vi "Impedance_SingleStats.vi"() -> ()   [LabVIEW 2020]
uses:
  <vilib>/Analysis/NI_AALBase.lvlib
panel:
  in  "Current Ch":tag="Dev3/ai1"
  in  "Voltage Ch":tag="Dev3/ai0"
  in  "Output channels":tag="Dev3/ao0"
  in  "TriggerLine":tag="/Dev3/ao/StartTrigger"
  out "Impedance (Phase) - AvgInput":dbl=-0.6720456229115541 format="%#_3p"
  out "Impedance (Mag) - AvgInput":dbl=100001.51067957297 format="%#_3p"
  out "Waveform Chart":dbl(graph)
  in  "Freq":dbl
  out "Histogram Graph Phase":T1(graph)
  out "Histogram Graph Mag":T1(graph)
  out "standard deviation  Z":dbl format="%.2p"
  out "standard deviation Phase":dbl format="%.2p"
  out "Real (Z) - AvgInput":dbl=0.483159362565652 format="%#_3p"
  out "Capacitance - AvgInput":dbl=-4.6875540145244966e-05 format="%#_3p"
  out "Inductance - AvgInput":dbl=5.4037341931629855e-06 format="%#_3p"
  out "Test Number":i32
  in  "Num Avg":i32=5
  out "Mean Phase":dbl format="%0.2f"
  out "Mean Mag":dbl format="%.4p"
  in  "amplitude":dbl=0.1 format="%0.2p"
  in  "SampRate":dbl=250000.0 format="%#.2p"
  in  "Test Time":dbl=1.0 format="%#_6p"
  in  "samples":i32=128
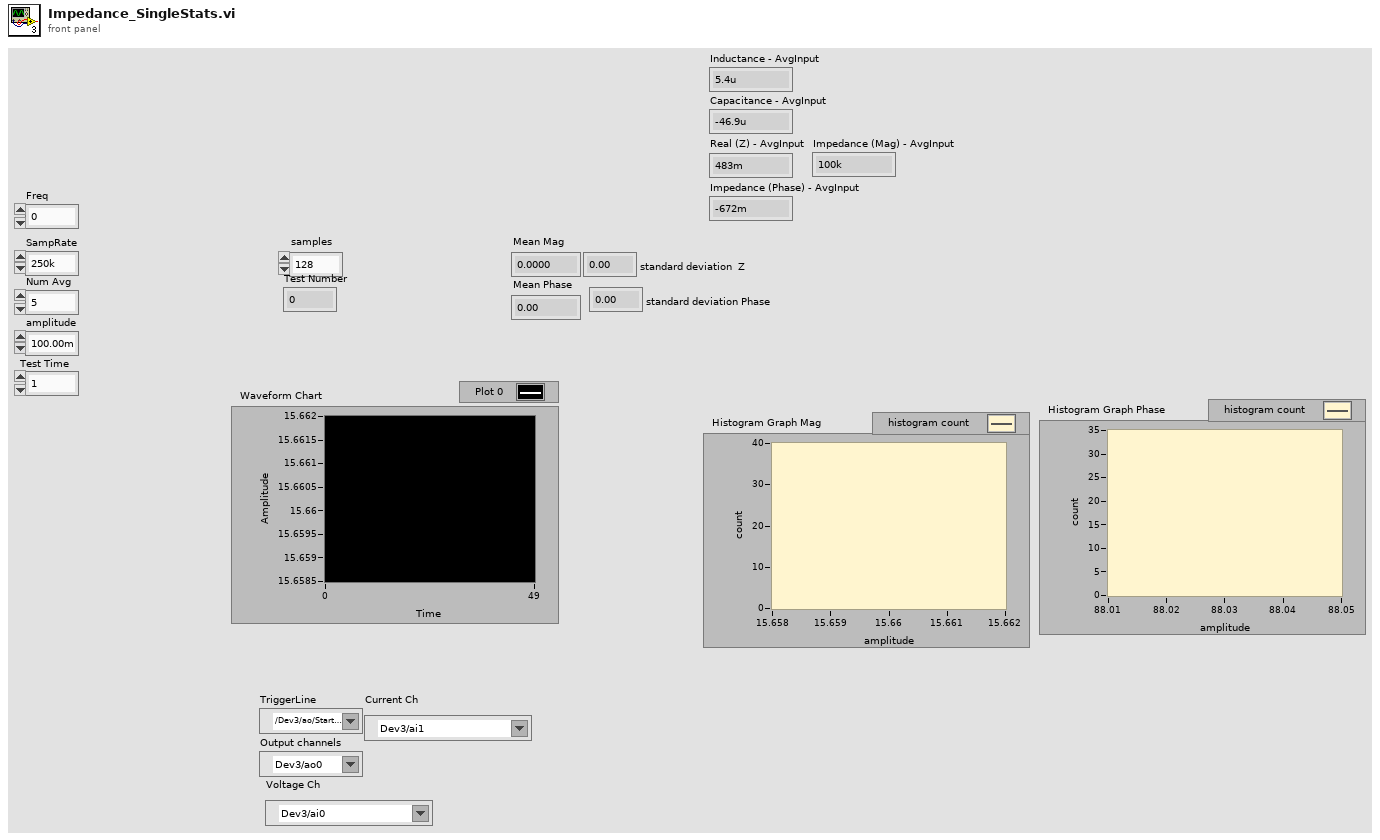
[diagram p1: front panel]
types:
  T1 = cluster{"X Values":dbl[], "Histogram: h(x)":i32[]}
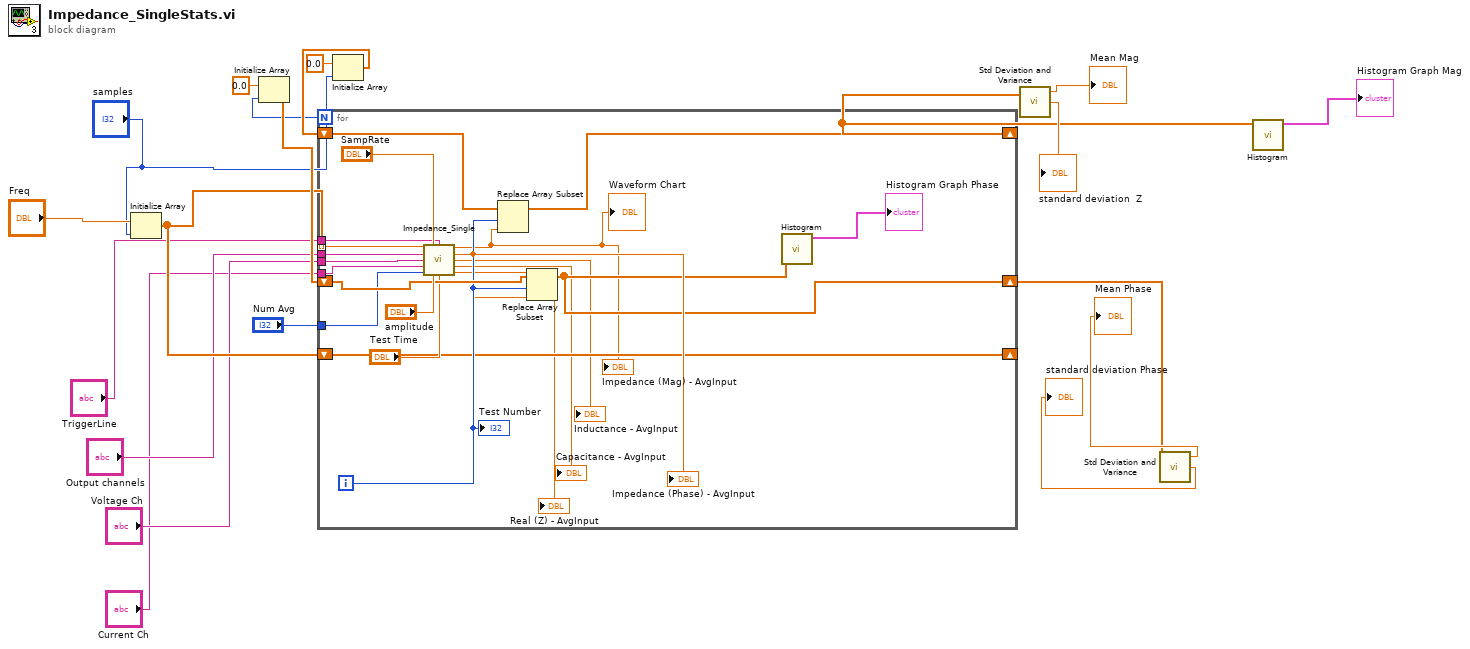
[diagram p0: block diagram]
diagram:
  n1 = Initialize Array("Freq", "samples") -> (w6:dbl[])
  n2 = Initialize Array(0.0 ("element"), "samples") -> (w16:dbl[])
  n3 = Initialize Array(0.0 ("element"), "samples") -> (w18:dbl[])
  n4 = for {
    N: "samples" -> [_]
    tunnel: w6 -> [w40] mode=indexing
    shift-right: [w27] -> w11
    shift-left: w18 -> [w39]
    shift-right: [w32] -> w9
    shift-left: w16 -> [w37]
    shift-right: [w31] -> _
    shift-left: w6 -> [w31]
    tunnel: "TriggerLine" -> [w24]
    tunnel: "Output channels" -> [w23]
    tunnel: "Voltage Ch" -> [w22]
    tunnel: "Current Ch" -> [w21]
    tunnel: "Num Avg" -> [w20]
    i -> [w36]
    n5 = call "Impedance_Single.vi"("Measure Frequency"=w40, "Sampling Rate"="SampRate", "TriggerLine"=w24, "Output channels"=w23, "Voltage Ch"=w22, "Current Ch"=w21, "Number of runs"=w20, "Amplitude (pk)"="amplitude", "Sampling Time"="Test Time") -> ("Impedance (Mag) - AvgInput"=w26:dbl, "Impedance (Phase) - AvgInput"=w35:dbl, "Inductance - AvgInput"=→"Inductance - AvgInput":dbl, "Capacitance - AvgInput"=→"Capacitance - AvgInput":dbl, "Real (Z) - AvgInput"=→"Real (Z) - AvgInput":dbl)  [unwired: 2 in]
    "Waveform Chart" <- w26
    "Impedance (Mag) - AvgInput" <- w26
    "Impedance (Phase) - AvgInput" <- w35
    n6 = Replace Array Subset(array=w39, new element=w26, index=w36) -> (w27:dbl[])
    n7 = Replace Array Subset(array=w37, new element=w35, index=w36) -> (w32:dbl[])
    n8 = call <vilib>:"Histogram.vi"("X"=w32) -> ("Histogram Graph"=→"Histogram Graph Phase":T1)  [unwired: 7 in, 3 out]
    "Test Number" <- w36
  }
  n9 = call <vilib>:"Std Deviation and Variance.vi"("X"=w11) -> ("mean"=→"Mean Mag":dbl, "standard deviation"=→"standard deviation  Z":dbl)  [unwired: 1 in, 1 out]
  n10 = call <vilib>:"Std Deviation and Variance.vi"("X"=w9) -> ("mean"=→"Mean Phase":dbl, "standard deviation"=→"standard deviation Phase":dbl)  [unwired: 1 in, 1 out]
  n11 = call <vilib>:"Histogram.vi"("X"=w11) -> ("Histogram Graph"=→"Histogram Graph Mag":T1)  [unwired: 7 in, 3 out]
